vi "Initialize.vi"(8 "error in (no error)":errorcluster, 9 "Reset (T: Reset)":bool=TRUE, 10 "ID Query (T: Check)":bool=TRUE, 11 "VISA resource name":refnum<visa-resource-name>) -> (0 "error out":errorcluster, 2 "Instrument Name":string, 3 "VISA resource name out":refnum<visa-resource-name>)   [LabVIEW 2020, in "Agilent 6XXX Series.lvlib"]
doc: "This VI passes the addressing information in the instrument decriptor to the Instr Open VI and returns the instrument ID. You can optionally reset the instrument by setting the front panel reset control. You must run this VI before using any of the instrument driver VIs for this instrument.\n\nThis driver supports the HP6030A, 6031A, 6032A, 6033A, 6035A, 6038A, 6621A, 6622A, 6623A, 6624A, 6627A, 6632A, 6633A, and the 6634A DC Power Supplies."
uses:
  <instrlib>/Agilent 6XXX Series/Agilent 6XXX Series.lvlib
panel:
  # "© 2005 National Instruments.  ALL RIGHTS RESERVED."
  # "Check\nDon't Check"
  # "Reset\nDon't Reset"
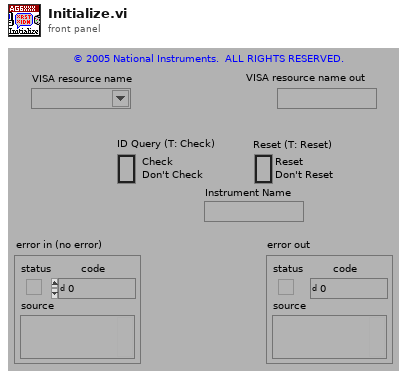
[diagram p1: front panel]
types:
  T1 = cluster{"status":bool, "code":i32, "VI name":string}
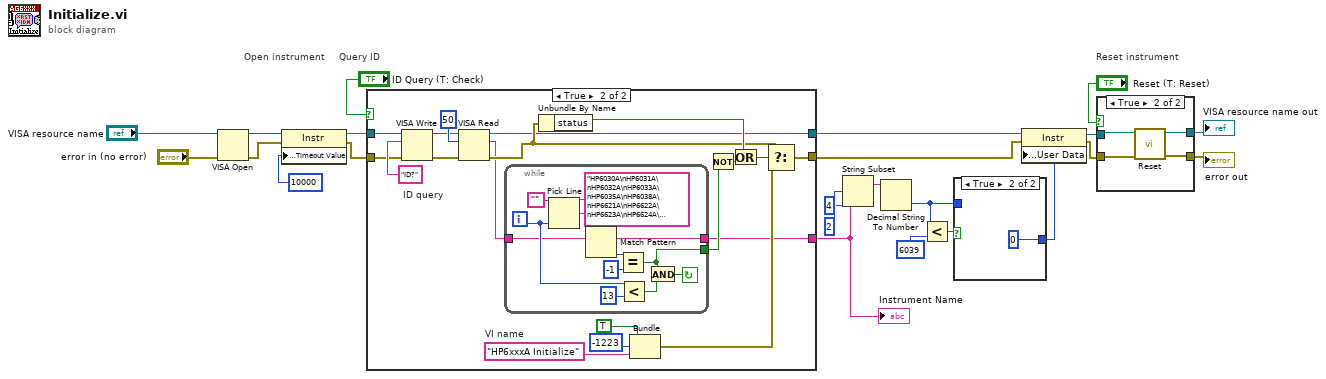
[diagram p0: block diagram]
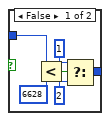
[diagram p2: hidden frame]
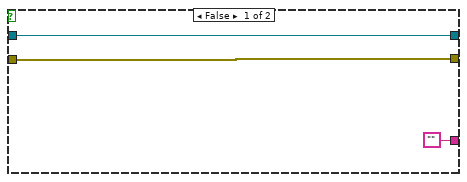
[diagram p4: hidden frame]
diagram:
  # "Query ID"
  # "Reset instrument"
  # "Open instrument"
  n1 = VISA Open(error in (no error)="error in (no error)", VISA resource name="VISA resource name") -> (VISA resource name=w5:refnum<visa-resource-name>, error out=w4:errorcluster)  [unwired: 3 in]
  n2 = property class="Instr"(reference=w5, error in=w4, "General Settings:Timeout Value"=u32 10000 ("Tmo Value")) -> (reference out=w2:refnum<visa-resource-name>, error out=w3:errorcluster)
  n3 = case shown="True" "ID Query (T: Check)" {
    tunnel: [w25 w31] -> w9
    tunnel: [w26 w34] -> w10
    tunnel: w2 -> [w26 w36]
    tunnel: w3 -> [w25 w39]
    tunnel: ["" w28] -> w18
    frame False {
    }
    frame True {
      w27 = "HP6xxxA Initialize"  # VI name
      w42 = "ID?"  # ID query
      n4 = VISA Write(VISA resource name=w36, write buffer=w42, error in (no error)=w39) -> (VISA resource name out=w35:refnum<visa-resource-name>, error out=w38:errorcluster)  [unwired: 1 out]
      n5 = VISA Read(VISA resource name=w35, byte count=u32 50, error in (no error)=w38) -> (VISA resource name out=w34:refnum<visa-resource-name>, read buffer=w33:string, error out=w37:errorcluster)  [unwired: 1 out]
      n6 = while {
        tunnel: [w46] -> w28
        tunnel: [w47] -> w29
        tunnel: w33 -> [w48]
        i -> [w52]
        stop <- w49 continue-if-true
        n7 = Pick Line(string ("")="", multi-line string="HP6030A\nHP6031A\nHP6032A\nHP6033A\nHP6035A\nHP6038A\nHP6621A\nHP6622A\nHP6623A\nHP6624A\nHP6627A\nHP6632A\nHP6633A\nHP6634A", line index=w52) -> (output string=w55:string)
        n8 = Match Pattern(string=w48, regular expression=w55) -> (match substring=w46:string, offset past match=w54:i32)  [unwired: 1 in, 2 out]
        n9 = Equal?(x=w54, y=-1) -> (x = y?=w47:bool)
        n10 = Less?(x=w52, y=13) -> (x < y?=w50:bool)
        n11 = And(x=w47, y=w50) -> (x .and. y?=w49:bool)
      }
      n12 = Unbundle By Name(w37) -> ("status"=w40:bool)
      n13 = Bundle(TRUE, -1223, "VI name"=w27) -> (w43:cluster{bool, i32, "VI name":string})  [unwired: 1 in]
      n14 = Not(x=w29) -> (.not. x?=w30:bool)
      n15 = Or(x=w40, y=w30) -> (x .or. y?=w32:bool)
      n16 = Select(t=w37, s=w32, f=w43) -> (s? t:f=w31:T1)
    }
  }
  "Instrument Name" <- w18
  n17 = String Subset(string=w18, offset (0)=2, length (rest)=4) -> (substring=w15:string)
  n18 = Decimal String To Number(string=w15) -> (number=w12:i32)  [unwired: 2 in, 1 out]
  n19 = Less?(x=w12, y=6039) -> (x < y?=w13:bool)
  n20 = case shown="True" w13 {
    tunnel: w12 -> [w62 _]
    tunnel: [w58 u32 0] -> w11
    frame False {
      n21 = Less?(x=w62, y=6628) -> (x < y?=w61:bool)
      n22 = Select(t=u32 1, s=w61, f=u32 2) -> (s? t:f=w58:u32)
    }
    frame True {
    }
  }
  n23 = property class="Instr"(reference=w10, error in=w9, "General Settings:User Data"=w11) -> (reference out=w7:refnum<visa-resource-name>, error out=w8:errorcluster)
  n24 = case shown="True" "Reset (T: Reset)" {
    tunnel: w8 -> [w66 w70]
    tunnel: [w66 w68] -> w20
    tunnel: w7 -> [w65 w69]
    tunnel: [w65 w67] -> w19
    frame False {
    }
    frame True {
      n25 = call <instrlib>:"Reset.vi"("error in (no error)"=w70, "VISA resource name"=w69) -> ("error out"=w68:errorcluster, "VISA resource name out"=w67:refnum<visa-resource-name>)  [unwired: 8 in]
    }
  }
  "VISA resource name out" <- w19
  "error out" <- w20
